vi "InitialiseDevice.vi"(8 "error In":errorcluster, 9 "PicoMotor IP In":string) -> (0 "error out":errorcluster, 1 "Device Address Out":i32, 2 "DeviceKey Out":string, 3 "CmdLib Out":refnum<k24>)   [LabVIEW 2013]
uses:
  C:/GEECS/Developers Version/source/Device Driver/Picomotor8742dotNet/NewFocus/CmdLib.dll
  CmdLib.dll
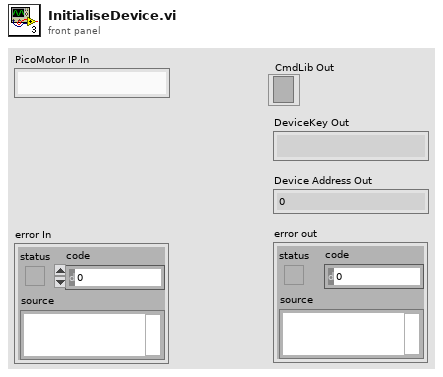
[diagram p1: front panel]
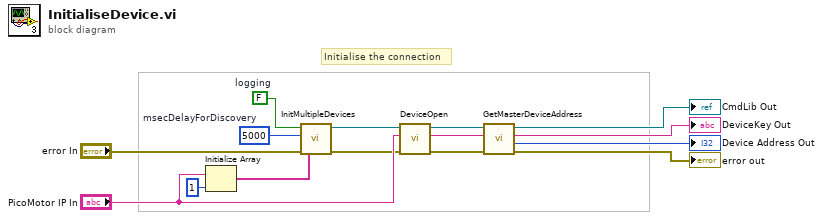
[diagram p0: block diagram]
diagram:
  w1 = FALSE  # logging
  w12 = 5000  # msecDelayForDiscovery
  # "Initialise the connection"
  n1 = Initialize Array("PicoMotor IP In", 1 ("dimension size")) -> (w11:string[])
  n2 = call "InitMultipleDevices.vi"("error in (no error)"="error In", "deviceKeys"=w11, "msecDelayForDiscovery"=w12, "logging"=w1) -> ("error out"=w7:errorcluster, "CmdLib Out"=w8:refnum<k24>)  [unwired: 1 in, 1 out]
  n3 = call "DeviceOpen.vi"("error in (no error)"=w7, "DeviceKey In"="PicoMotor IP In", "CmdLib In"=w8) -> ("error out"=w13:errorcluster, "DeviceKey Out"=w14:string, "CmdLib Out"=w15:refnum<k24>)  [unwired: 2 in]
  n4 = call "GetMasterDeviceAddress.vi"("error in (no error)"=w13, "DeviceKey In"=w14, "CmdLib In"=w15) -> ("error out"=→"error out":errorcluster, "Device Address"=→"Device Address Out":i32, "DeviceKey Out"=→"DeviceKey Out":string, "CmdLib Out"=→"CmdLib Out":refnum<k24>)  [unwired: 1 in]
